vi "queryError.vi"(8 "error in (no error)":errorcluster, 11 "ElectrometerController in":refnum<class "ElectrometerController.lvclass">) -> (0 "error out":errorcluster, 2 "ErrorArray":T1[](array[typedef]), 3 "ElectrometerController out":refnum<class "ElectrometerController.lvclass">)   [LabVIEW 2016, in "ElectrometerController.lvclass"]
uses:
  ElectrometerController.lvclass
  ElectrometerError/Controls/errorType.ctl
  Electrometer/Electrometer.lvclass
  ElectrometerError/ElectrometerError.lvclass
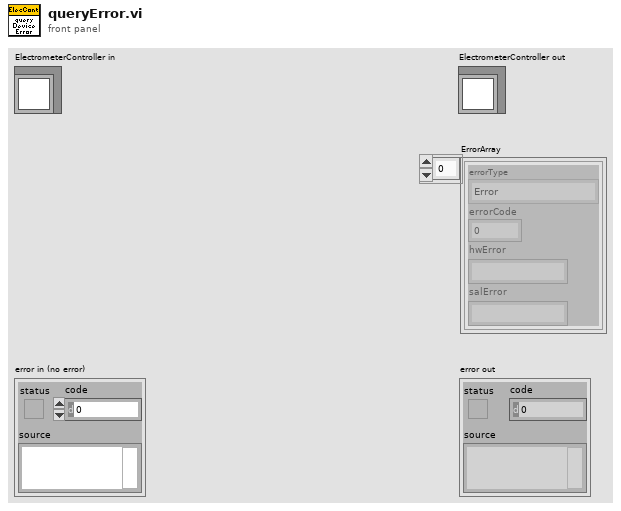
[diagram p1: front panel]
types:
  T1 = typedef "ElectrometerError.lvclass/errorType.ctl" = cluster{"errorType":enum16{"Error", "Warning", "None"}, "errorCode":dbl, "hwError":string, "salError":string}
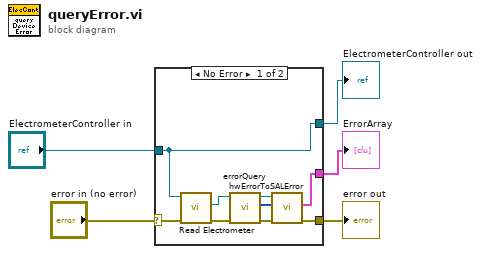
[diagram p0: block diagram]
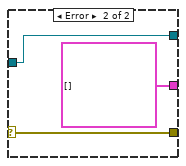
[diagram p2: hidden frame]
diagram:
  n1 = case shown="No Error" "error in (no error)" {
    selector: "error in (no error)" -> [w12 w17]
    tunnel: [w9 w17] -> w4
    tunnel: [w14 w16] -> w2
    tunnel: "ElectrometerController in" -> [w14 w16]
    tunnel: [w6 T1[] [] ("ErrorArray")] -> w1
    frame No Error {
      n2 = call-dynamic "Read Electrometer.vi"("error in (no error)"=w12, "ElectrometerController in"=w14) -> ("error out"=w13:errorcluster, "Electrometer.lvclass"=w11:refnum<class "Electrometer.lvclass">)  [unwired: 7 in, 1 out]
      n3 = call "errorQuery.vi"("error in (no error)"=w13, "Electrometer in"=w11) -> ("error out"=w10:errorcluster, "Device Error"=w7:i32[], "Electrometer out"=w8:refnum<class "Electrometer.lvclass">)  [unwired: 6 in, 1 out]
      n4 = call-dynamic "hwErrorToSALError.vi"("error in (no error)"=w10, "Error Code"=w7, "Electrometer in"=w8) -> ("error out"=w9:errorcluster, "ErrorArray"=w6:T1[])  [unwired: 6 in, 1 out]
    }
    frame Error {
    }
  }
  "error out" <- w4
  "ElectrometerController out" <- w2
  "ErrorArray" <- w1
